vi "ProdaNG.TestStepResult.New.vi"(8 "error in (no error)":errorcluster, 10 "TestStepResult":T1, 11 "dbHandle":i32) -> (0 "error out":errorcluster, 2 "TestStepResult out":T1, 3 "dbHandle":i32)   [LabVIEW 2016]
doc: "This function creates a new record from a prefilled TestStepResult structure. Additionally the mdTime in the according product is set the current time.\nParameter:\nhandle is an Integer, which is returned by the function Login() at the creation of a new connection.\ntestStepResult is a pointer on a TestStepResult structure, which elements must be prefilled. The structure must be defined and filled in the calling program. Nearly all elements of the structure must be set to reasonable values. The element id is filled by the DLL with a new Id for the created record, if the returncode is 0.\nThe element statusId is of particular importance:\nIf this element is passed with the value -1, the DLL automatically sets the standard status 2 (in Process), while otherwise the returned status is set.\n\nReturncodes:\n0 No error \n< 0 ORACLE Error code\n 6 (ERROR_INVALID_HANDLE) in case of an invalid handle"
uses:
  Controls/ProdaNG.TestStepResult.ctl
  Controls/ProdaNG.TestStepResultSize.ctl
  prodllNG.dll
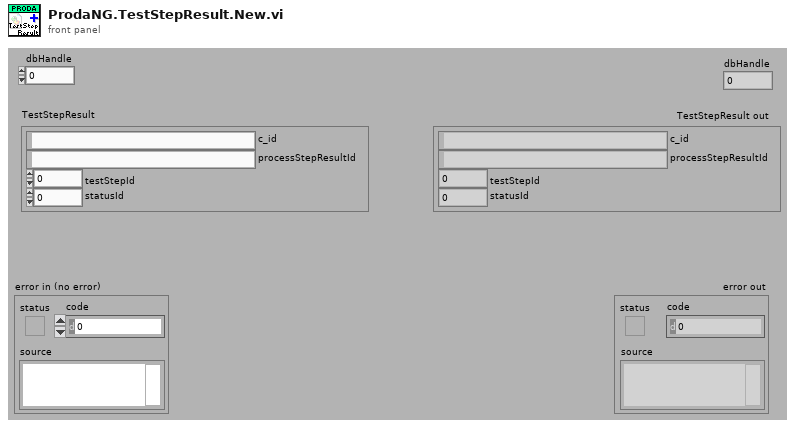
[diagram p1: front panel]
types:
  T1 = typedef "ProdaNG.TestStepResult.ctl" = cluster{"c_id":string, "processStepResultId":string, "testStepId":i32, "statusId":i32}
  T2 = typedef "ProdaNG.TestStepResultSize.ctl" = cluster{"c_id":i32, "processStepResultId":i32, "testStepId":i32, "statusId":i32}
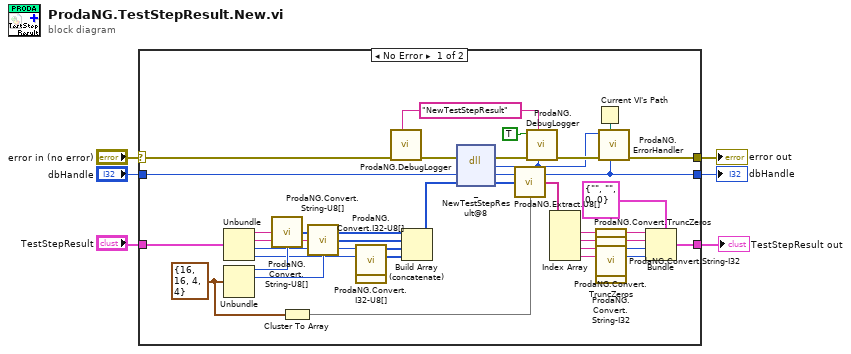
[diagram p0: block diagram]
diagram:
  n1 = case shown="No Error" "error in (no error)" {
    selector: "error in (no error)" -> [w13 w46]
    tunnel: [w11 w46] -> w5
    tunnel: "dbHandle" -> [w12 w45]
    tunnel: [w10 w45] -> w3
    tunnel: [w9 w44] -> w2
    tunnel: "TestStepResult" -> [w8 w44]
    frame No Error {
      w7 = T2 {"c_id"=16, "processStepResultId"=16, "testStepId"=4, "statusId"=4} ("TestStepResultSize")
      w40 = "NewTestStepResult" ("cmd")
      n2 = Unbundle(w8) -> ("c_id"=w42:string, "processStepResultId"=w43:string, "testStepId"=w30:i32, "statusId"=w29:i32)
      n3 = Unbundle(w7) -> ("c_id"=w34:i32, "processStepResultId"=w32:i32)  [unwired: 2 out]
      n4 = call "ProdaNG.Convert.String-U8[].vi"("Input String"=w42, "Size"=w34) -> ("Output"=w33:u8[])
      n5 = Cluster To Array(cluster=w7) -> (array=w17:i32[])
      n6 = call "ProdaNG.Convert.String-U8[].vi"("Input String"=w43, "Size"=w32) -> ("Output"=w31:u8[])
      n7 = call "ProdaNG.Convert.I32-U8[].vi"("32bit integer"=w30) -> ("unsigned byte array"=w28:u8[])  [unwired: 10 in]
      n8 = call "ProdaNG.Convert.I32-U8[].vi"("32bit integer"=w29) -> ("unsigned byte array"=w27:u8[])  [unwired: 10 in]
      n9 = call "ProdaNG.DebugLogger.vi"("cmd"=w40, "error in (no error)"=w13) -> ("error out"=w35:errorcluster)  [unwired: 9 in]
      n10 = Build Array (concatenate)(w33, w31, w28, w27) -> (w26:u8[])
      n11 = dll-call lib="D:/svn/LineTraceSystem/SOFTWARE/sources/Database/ProdaNG/prodllNG.dll" fn="_NewTestStepResult@8" ("ProDll.dll:InitProDll")(error in=w35, "dbHandle"=w12, "testStepResult"=w26) -> (error out=w38:errorcluster, "return type"=w36:i32, "dbHandle"=w10:i32, "testStepResult"=w18:u8[])  [unwired: 2 in, 1 out]
      n12 = call "ProdaNG.Extract.U8[].vi"("unsigned byte array"=w18, "Sizes"=w17) -> ("Elements"=w16:string[])
      n13 = call "ProdaNG.DebugLogger.vi"("return type"=w36, "cmd"=w40, "error in (no error)"=w38, "done? (F)"=TRUE) -> ("error out"=w37:errorcluster)  [unwired: 7 in]
      n14 = Index Array(array=w16) -> (element #1=w20:string, element #2=w19:string, element #3=w25:string, element #4=w14:string)  [unwired: 4 in]
      n15 = Current VI's Path() -> (path=w41:path)
      n16 = call "ProdaNG.Convert.TruncZeros.vi"("string with \\0s"=w20) -> ("LV string"=w22:string)  [unwired: 10 in]
      n17 = call "ProdaNG.Convert.TruncZeros.vi"("string with \\0s"=w19) -> ("LV string"=w21:string)  [unwired: 10 in]
      n18 = call "ProdaNG.Convert.String-I32.vi"("unsigned byte string"=w25) -> ("32bit integer"=w24:i32)  [unwired: 10 in]
      n19 = call "ProdaNG.Convert.String-I32.vi"("unsigned byte string"=w14) -> ("32bit integer"=w23:i32)  [unwired: 10 in]
      n20 = call "ProdaNG.ErrorHandler.vi"("dbHandleIn"=w10, "Path"=w41, "error in"=w37, "output_parameter"=w36) -> ("error out"=w11:errorcluster)  [unwired: 7 in]
      n21 = Bundle(cluster=T1 {"c_id"="", "processStepResultId"="", "testStepId"=0, "statusId"=0} ("ProcessStepResult out"), "c_id"=w22, "processStepResultId"=w21, "testStepId"=w24, "statusId"=w23) -> (w9:T1)
    }
    frame Error {
    }
  }
  "error out" <- w5
  "dbHandle" <- w3
  "TestStepResult out" <- w2
